vi "cv_05_clusters.vi"() -> ()   [LabVIEW 2013]
panel:
  in  "String 2":string
  out "OUT Cluster 2":T1
  in  "IN Cluster 2":T1
  in  "String":string
  out "OUT Cluster":T1
  in  "IN Cluster":T1
  in  "Cluster":T2
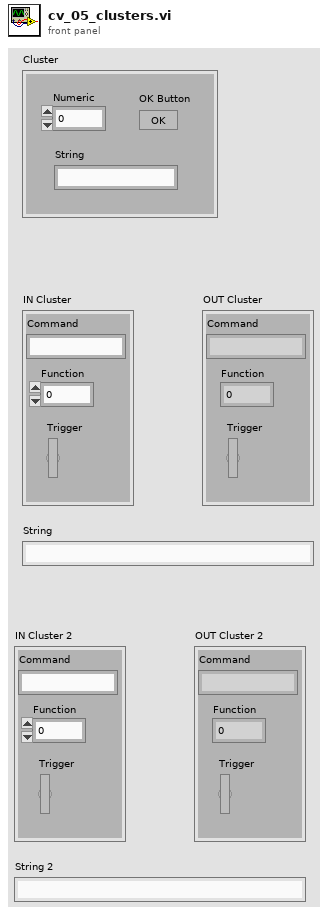
[diagram p1: front panel]
types:
  T1 = cluster{"Command":string, "Function":dbl, "Trigger":bool}
  T2 = cluster{"Numeric":dbl, "OK Button":bool, "String":string}
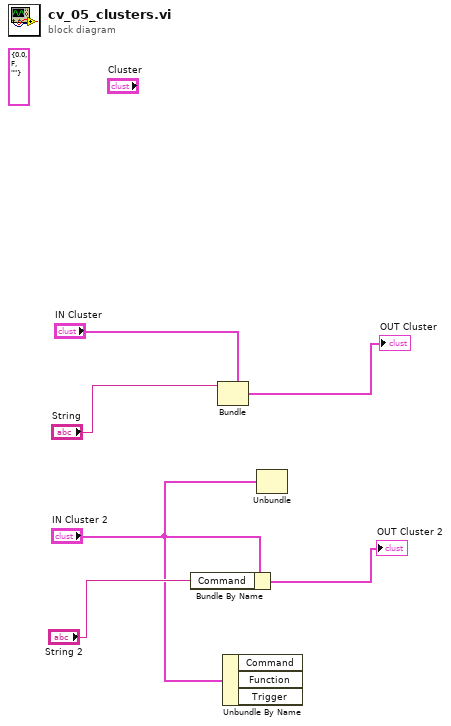
[diagram p0: block diagram]
diagram:
  (unwired) T2 {"Numeric"=0.0, "OK Button"=FALSE, "String"=""} ("Cluster")
  n1 = Bundle By Name(cluster="IN Cluster 2", "Command"="String 2") -> (→"OUT Cluster 2":T1)
  n2 = Bundle(cluster="IN Cluster", "Command"="String") -> (→"OUT Cluster":T1)  [unwired: 2 in]
  n3 = Unbundle By Name("IN Cluster 2") -> ()  [unwired: 3 out]
  n4 = Unbundle("IN Cluster 2") -> ()  [unwired: 3 out]
